vi "Unbundle.vi"(8 "error in":errorcluster, 11 "Instrument Alias Data in":refnum<class "Instrument Alias Data.lvclass">) -> (0 "error out":errorcluster, 2 "Instrument Info Array":T1[](array[typedef]), 3 "Instrument Alias Data out":refnum<class "Instrument Alias Data.lvclass">)   [LabVIEW 2020, in "Instrument Handler.lvlib" / "Instrument Alias Data.lvclass"]
doc: "Read the Instrument Alias Data."
uses:
  Instrument Alias Data.lvclass
  Controls/Ctl_DriverAliasElement.ctl
  Instrument Alias Data.lvclass/Instrument Alias Data.ctl
  Instrument Handler.lvlib
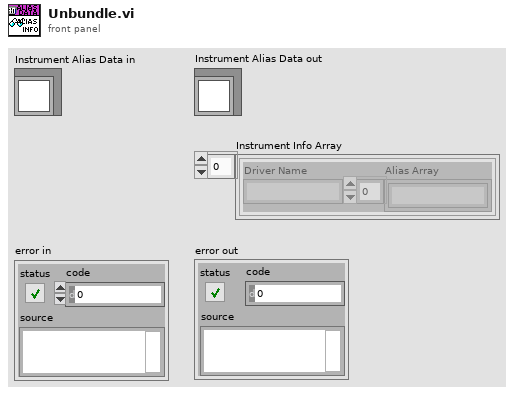
[diagram p1: front panel]
types:
  T1 = typedef "Instrument Handler.lvlib/Ctl_DriverAliasElement.ctl" = cluster{"Driver Name":string, "Alias Array":string[]}
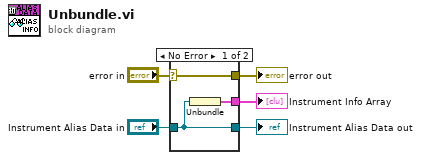
[diagram p0: block diagram]
diagram:
  n1 = case shown="No Error" "error in" {
    selector: "error in" -> [w7 w9]
    tunnel: [w6 w10] -> w5
    tunnel: "Instrument Alias Data in" -> [w6 w10]
    tunnel: [w8 _] -> w3
    tunnel: [w7 w9] -> w1
    frame No Error {
      n2 = Unbundle(w6) -> (w8:T1[])
    }
    frame Error {
    }
  }
  "Instrument Alias Data out" <- w5
  "Instrument Info Array" <- w3
  "error out" <- w1
